vi "checklist_popup.vi"(11 "Session Checklist In":T1) -> (3 "Session Checklist Out":T1)   [LabVIEW 2013]
uses:
  MouseCarousel/Checklists/SessionChecklist.ctl
panel:
  in  "Stop":bool
  in  "Check All Btn":bool
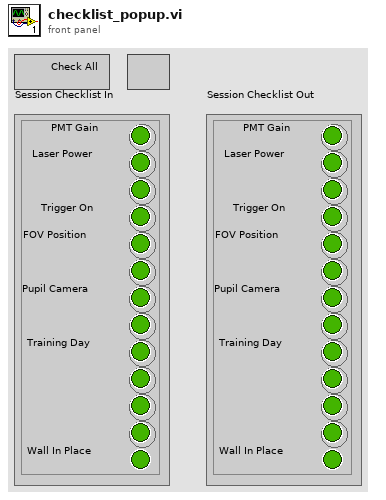
[diagram p1: front panel]
types:
  T1 = typedef "SessionChecklist.ctl" = cluster{"PMT Gain":bool, "Laser Power":bool, "Experiment Name":bool, "Trigger On":bool, "FOV Position":bool, "Security Camera":bool, "Pupil Camera":bool, "Pupil Cropped":bool, "Training Day":bool, "Closed Curtain":bool, "Lights On/Off":bool, "Lickport In Place":bool, "Wall In Place":bool}
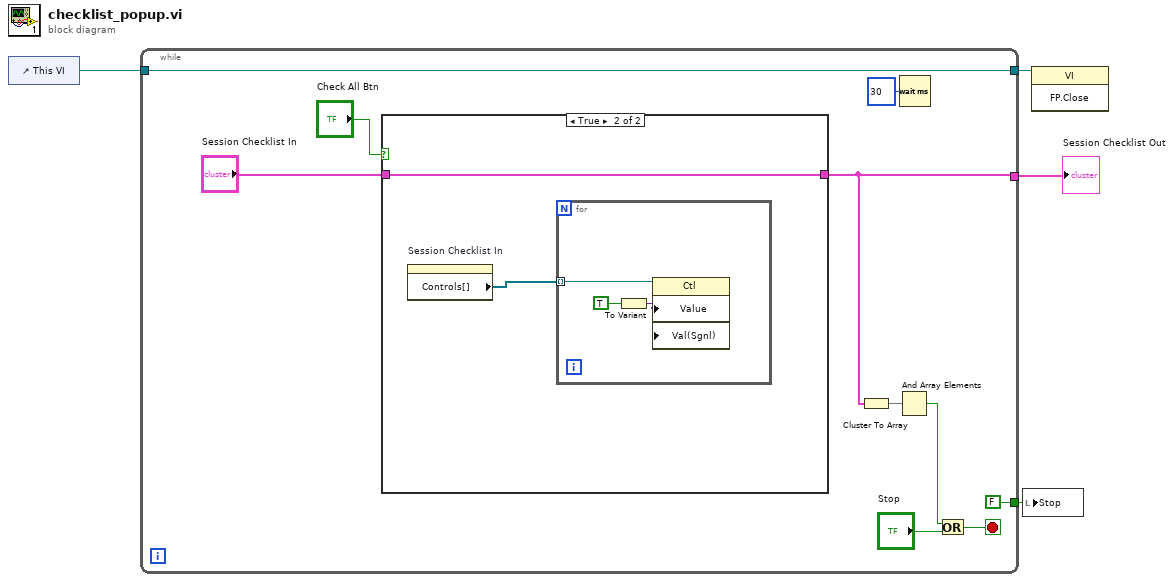
[diagram p0: block diagram]
diagram:
  n1 = control-ref of="This VI"() -> (w2:refnum<vi>)
  n2 = while {
    tunnel: [w9] -> w4
    tunnel: [FALSE] -> w3
    tunnel: w2 -> [w5]
    tunnel: [w5] -> w1
    stop <- w12 stop-if-true
    n3 = case shown="True" "Check All Btn" {
      tunnel: "Session Checklist In" -> [w15 w17]
      tunnel: [w15 w17] -> w9
      frame False {
      }
      frame True {
        n4 = property on="Session Checklist In" class="Clust (strict)"() -> ("Controls[]"=w16:refnum<vi>[])  [unwired: 2 in, 2 out]
        n5 = for {
          tunnel: w16 -> [w19] mode=indexing
          n6 = To Variant(anything=TRUE) -> (Variant=w18:variant)
          n7 = property class="Ctl"(reference=w19, "Value"=w18, "Val(Sgnl)"=w18) -> ()  [unwired: 1 in, 2 out]
        }
      }
    }
    n8 = Cluster To Array(cluster=w9) -> (array=w10:bool[])
    n9 = And Array Elements(Boolean array=w10) -> (logical AND=w11:bool)
    n10 = Wait (ms)(milliseconds to wait=u32 30) -> ()  [unwired: 1 out]
    n11 = Or(x=w11, y="Stop") -> (x .or. y?=w12:bool)
  }
  "Session Checklist Out" <- w4
  n12 = local write "Stop"(w3) -> ()
  n13 = invoke class="VI" method="FP.Close"(reference=w1) -> ()  [unwired: 2 in, 3 out]
